vi "Andor_ShutdownBox.vi"() -> ()   [LabVIEW 2018]
panel:
  in  "Close":bool
  out "Current temperature":i32
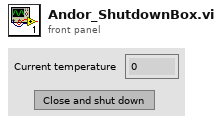
[diagram p1: front panel]
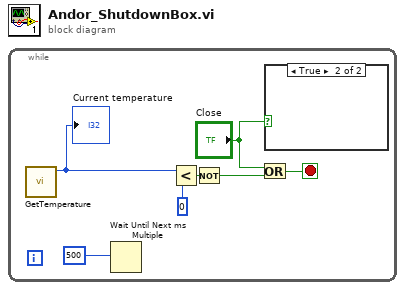
[diagram p0: block diagram]
diagram:
  n1 = while {
    stop <- w4 stop-if-true
    n2 = call <userlib>:"GetTemperature.vi"() -> ("temperature"=w1:i32)  [unwired: 4 in, 3 out]
    "Current temperature" <- w1
    n3 = Wait Until Next ms Multiple(millisecond multiple=u32 500) -> ()  [unwired: 1 out]
    n4 = Less?(x=w1, y=i16 0) -> (x < y?=w6:bool)
    n5 = Not(x=w6) -> (.not. x?=w3:bool)
    n6 = Or(x="Close", y=w3) -> (x .or. y?=w4:bool)
    n7 = case shown="True" "Close" {
      frame False {
      }
      frame True {
      }
    }
  }
